vi "XML Script - Append Terminal Name (Shift Register -  Right).vi"(1 "shiftreg":string) -> (0 "shiftreg.Right":string)   [LabVIEW 2017]
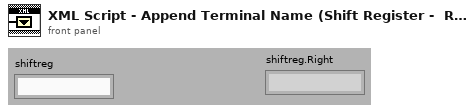
[diagram p1: front panel]
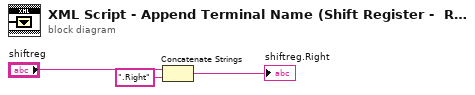
[diagram p0: block diagram]
diagram:
  n1 = Concatenate Strings("shiftreg", ".Right" ("string")) -> (→"shiftreg.Right":string)
